vi "Setup.vi"(11 "jettl Msg Setup in":refnum<class "jettl Msg Setup.lvclass">) -> (3 "jettl Msg Setup out":refnum<class "jettl Msg Setup.lvclass">)   [LabVIEW 2021, in "Setup Msg Strategy.lvlib" / "jettl Msg Setup.lvclass"]
uses:
  jettl Msg Setup.lvclass
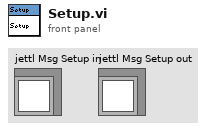
[diagram p1: front panel]
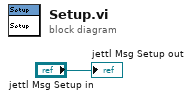
[diagram p0: block diagram]
diagram:
  "jettl Msg Setup out" <- "jettl Msg Setup in"
